vi "Actor Core.vi"(8 "error in":errorcluster, 11 "Controller Actor in":refnum<class "Controller Actor.lvclass">) -> (0 "error out":errorcluster, 3 "Controller Actor out":refnum<class "Actor.lvclass">)   [LabVIEW 2016, in "Event Actors.lvlib" / "Controller Actor.lvclass"]
doc: "(<B>Filename</B>: Actor Framework.lvlib:Actor.lvclass:Actor Core.vi)\n\nReceives messages to the actor, reacts to them, and initiates any error handling that may shut the actor down.\n\nDescendant classes may override this VI to append parallel tasks for the actor to complete while it handles messages. Overrides use the Call Parent Method node."
uses:
  Controller Actor.lvclass
  <vilib>/ActorFramework/Actor/Actor.lvclass
  <vilib>/MGI/Monitored Actor/Monitored Actor/Monitored Actor/Monitored Actor.lvclass
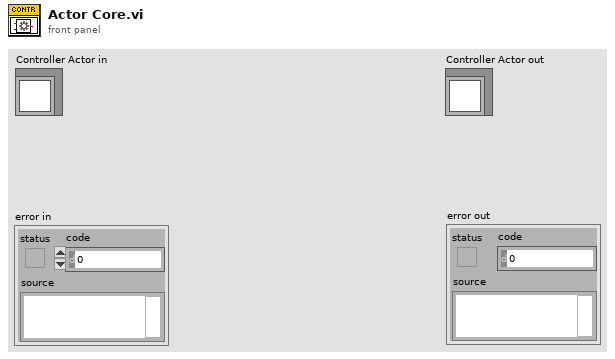
[diagram p1: front panel]
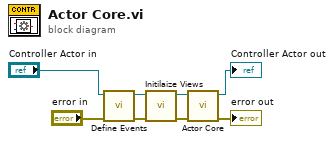
[diagram p0: block diagram]
diagram:
  n1 = call-dynamic "Define Events.vi"("error in (no error)"="error in", "Controller Actor in"="Controller Actor in") -> ("error out"=w2:errorcluster, "Controller Actor out"=w1:refnum<class "Controller Actor.lvclass">)  [unwired: 8 in]
  n2 = call-dynamic "Initilaize Views.vi"("error in (no error)"=w2, "Controller Actor in"=w1) -> ("error out"=w3:errorcluster, "Controller Actor out"=w5:refnum<class "Controller Actor.lvclass">)  [unwired: 8 in]
  n3 = call-parent "Actor Core.vi"("error in"=w3, "Actor in"=w5) -> ("error out"=→"error out":errorcluster, "Actor out"=→"Controller Actor out":refnum<class "Actor.lvclass">)  [unwired: 8 in]
